vi "VNA and Opticool.vi"() -> ()   [LabVIEW 2022 SP3]
uses:
  <vilib>/Analysis/baseanly.llb/Mean (DBL).vi
  <vilib>/Utility/file.llb/Write Delimited Spreadsheet (DBL).vi
  <vilib>/Analysis/NI_AALBase.lvlib
  Agilent ENA Series/Agilent ENA Series.lvlib
panel:
  in  "stop":bool
  in  "file path (dialog if empty) Scan 2":path=path "C:/Users/B1172_SHG/Documents/NOEMS/test.txt"
  in  "Second Scan":bool
  in  "Port ( 1)  2":i32=1
  in  "Measurement Parameters   2":u16(ring)=1 items=["S11", "S21", "S31", "S41", "S12", "S22", "S32", "S42", "S13", "S23", "S33", "S43", "S14", "S24", "S34", "S44", "A", "B", "C", "D", "R1", "R2", "R3", "R4"]
  in  "Power Level (dBm)  2":dbl=-5.0 format="%^.2g"
  in  "VNA Points  2":i32=1000
  in  "Start (Mhz)  2":dbl=1.0 format="%^.2e"
  in  "Stop (MHz)  2":dbl=10.0 format="%^.2e"
  in  "Trigger Source   2":u16(ring) items=["Internal", "External", "Manual", "BUS"]
  in  "Point Trigger (F: Disable) 3":bool
  in  "Continuous Sweep (T: Enable)  2":bool=TRUE
  in  "Averaging State (F: Off) 3":bool
  in  "Average Factor (16) 3":i32=16
  in  "IF Bandwidth (100000.0)  2":dbl=1000.0 format="%^.1e"
  in  "Smoothing State (F: Off) 3":bool
  in  "Wait time (ms)  2":dbl=4000.0
  out "XY Graph 3":cluster{dbl[], "Primary / Real":dbl[]}(graph)
  in  "Continue":bool
  in  "Field Set when finsihed":dbl
  in  "Port ( 1)":i32=1
  in  "Measurement Parameters":u16(ring)=1 items=["S11", "S21", "S31", "S41", "S12", "S22", "S32", "S42", "S13", "S23", "S33", "S43", "S14", "S24", "S34", "S44", "A", "B", "C", "D", "R1", "R2", "R3", "R4"]
  in  "Power Level (dBm)":dbl=-5.0 format="%^.2g"
  in  "VNA Points":i32=1000
  in  "Start (Mhz)":dbl=1.0 format="%^.2e"
  in  "Stop (MHz)":dbl=10.0 format="%^.2e"
  in  "Trigger Source":u16(ring) items=["Internal", "External", "Manual", "BUS"]
  in  "Point Trigger (F: Disable) 2":bool
  in  "Continuous Sweep (T: Enable)":bool=TRUE
  in  "Averaging State (F: Off) 2":bool
  in  "Average Factor (16) 2":i32=16
  in  "IF Bandwidth (100000.0)":dbl=1000.0 format="%^.1e"
  in  "Smoothing State (F: Off) 2":bool
  in  "Wait time (ms)":dbl=4000.0
  out "XY Graph 2":cluster{dbl[], "Primary / Real":dbl[]}(graph)
  in  "T scan waiting time (min)":dbl=20.0
  in  "Scan T":bool=TRUE
  in  "T Step Size":dbl
  in  "Start B":dbl
  in  "B Step Size":dbl
  in  "B Number of Step":i32=1
  in  "Start T":dbl
  in  "T Number of Step":i32=1
  in  "Temperature Set when finish":dbl=120.0
  in  "file path (dialog if empty)":path=path "C:/Users/B1172_SHG/Documents/NOEMS/test.txt"
  in  "VISA resource name":refnum<visa-resource-name>
  in  "Remote":bool=TRUE
  in  "IP Address":string="169.254.170.239"
  out "Measuring":bool
  out "Temperature":dbl
  in  "WaitForTemperature":bool=TRUE
  in  "WaitForField":bool=TRUE
  in  "Delay":dbl=5.0
  out "Field":dbl
  out "Field\nStatus":i32(ring) items=["MagnetUnknown"=0, "StablePersistent"=1, "WarmingSwitch"=2, "CoolingSwitch"=3, "StableDriven"=4, "Iterating"=5, "Charging"=6, "Discharging"=7, "CurrentError"=8, "MagnetFailure"=15]
  out "Temperature\nStatus":i32(ring) items=["TemperatureUnknown"=0, "Stable"=1, "Tracking"=2, "Near"=5, "Chasing"=6, "Filling"=7, "Standby"=10, "Disabled"=13, "ImpedanceNotFunction"=14, "TempFailure"=15]
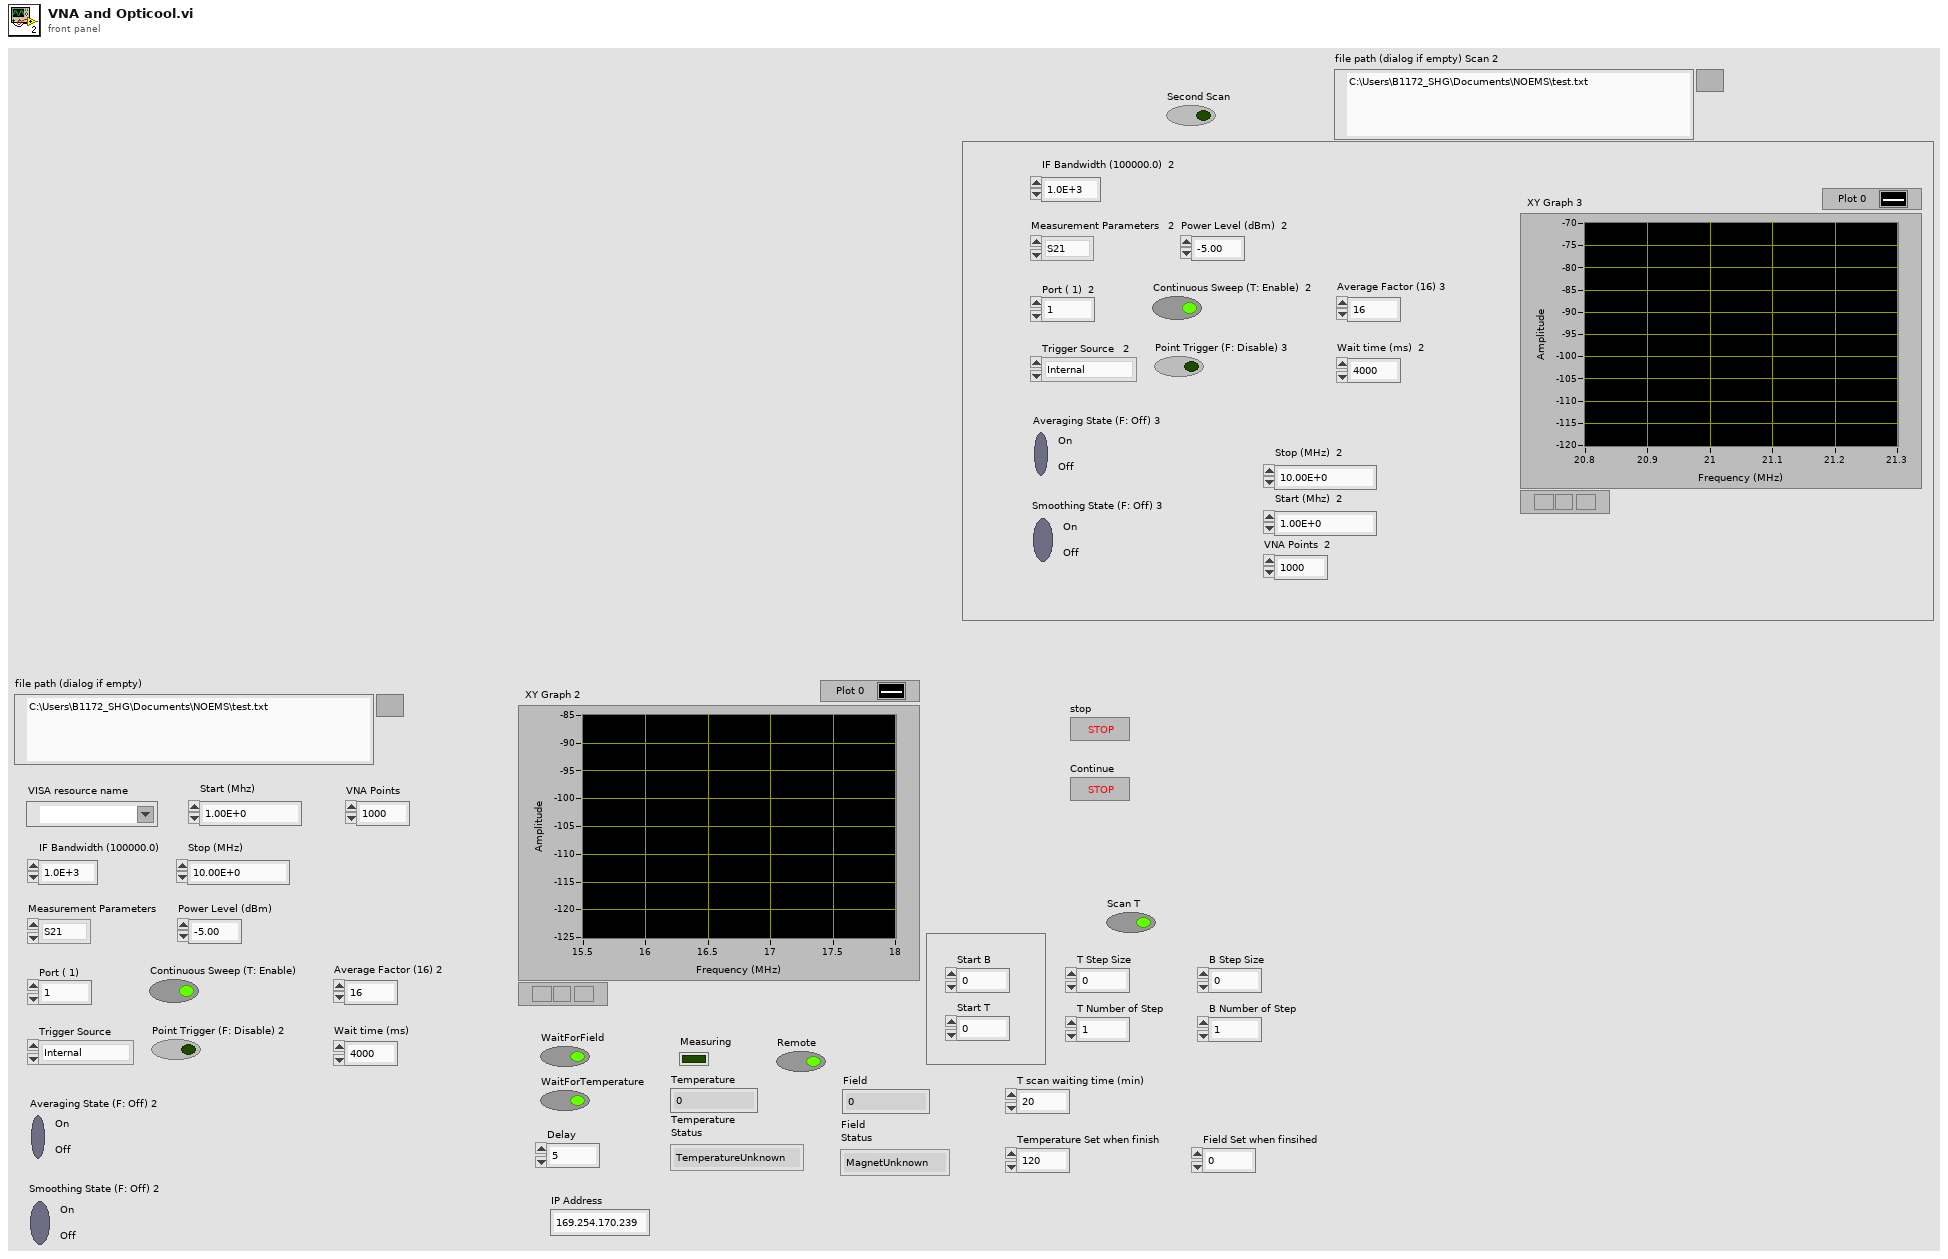
[diagram p1: front panel]
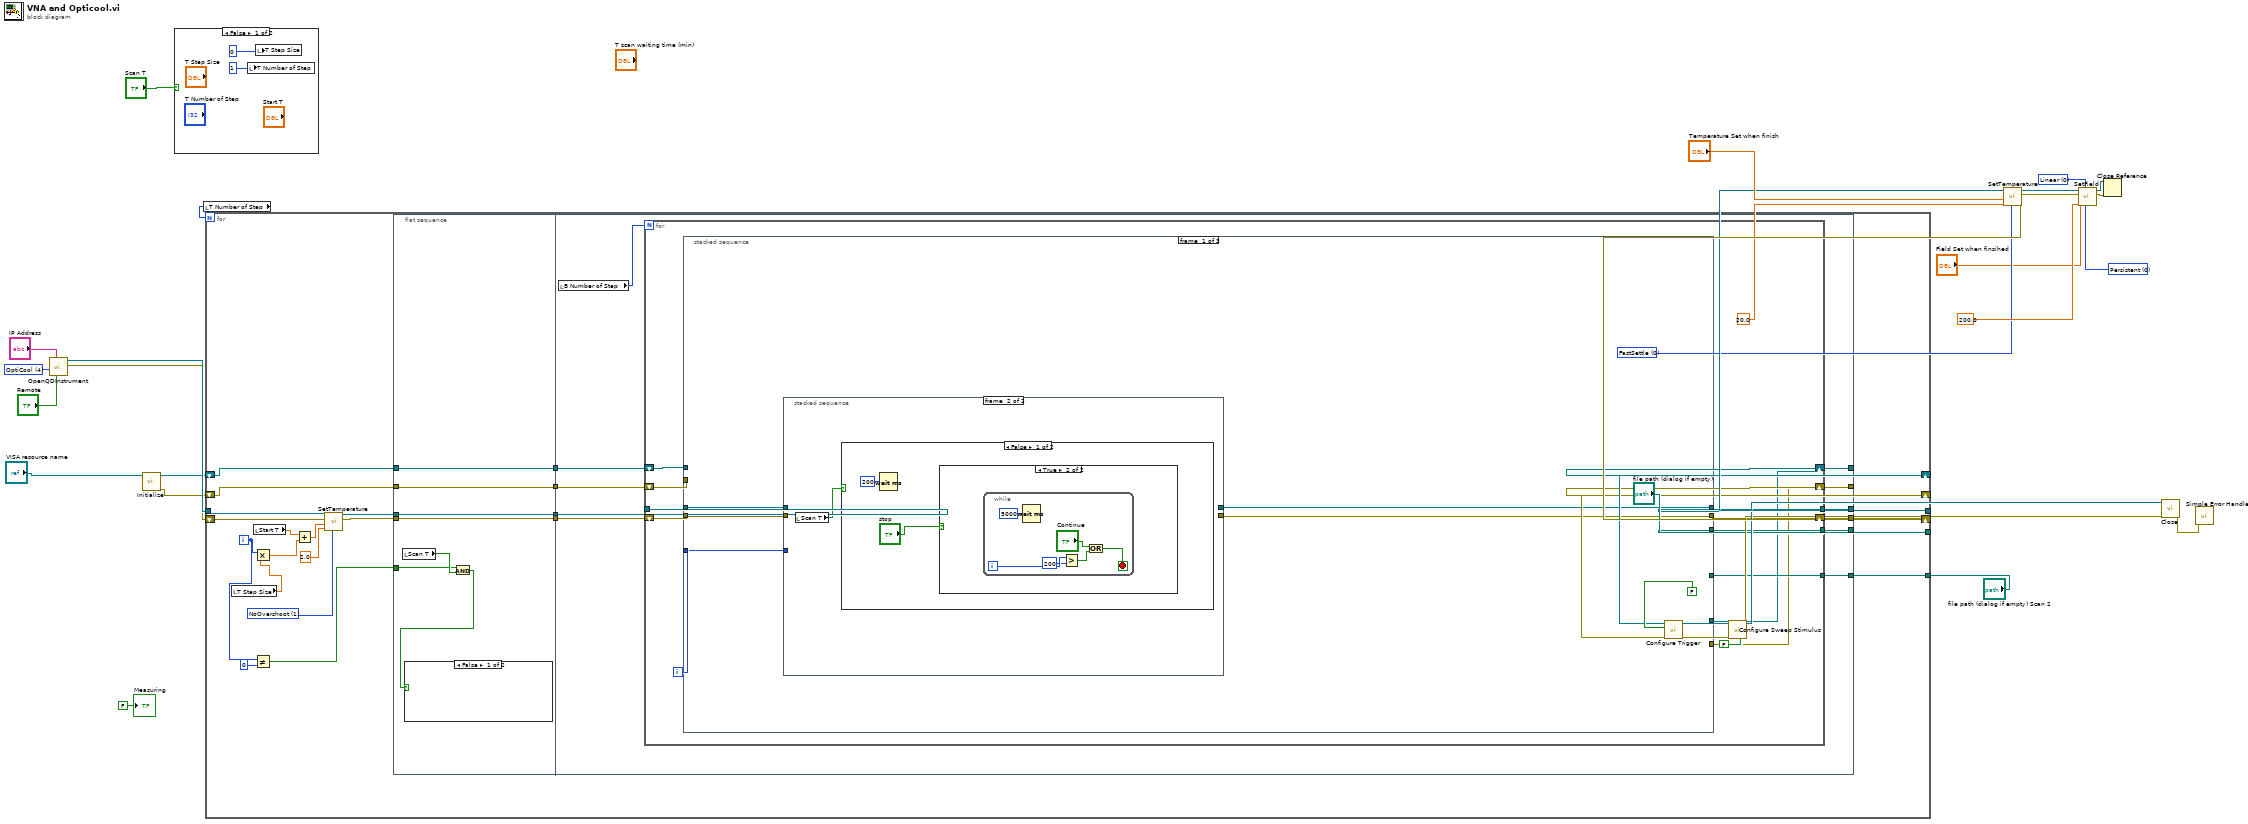
[diagram p0: block diagram]
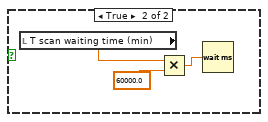
[diagram p2: hidden frame]
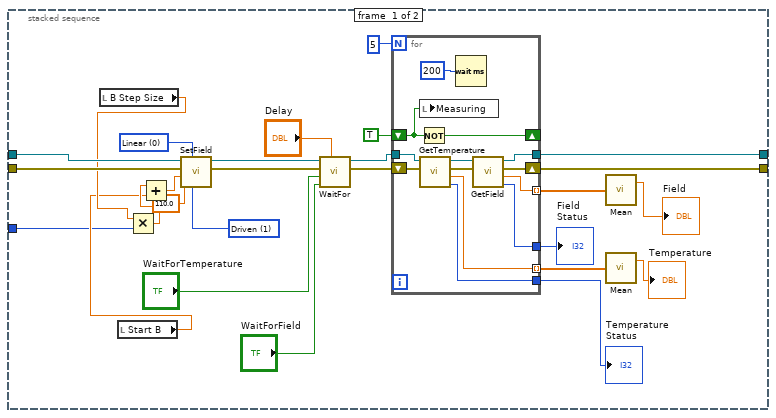
[diagram p3: hidden frame]
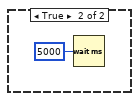
[diagram p5: hidden frame]
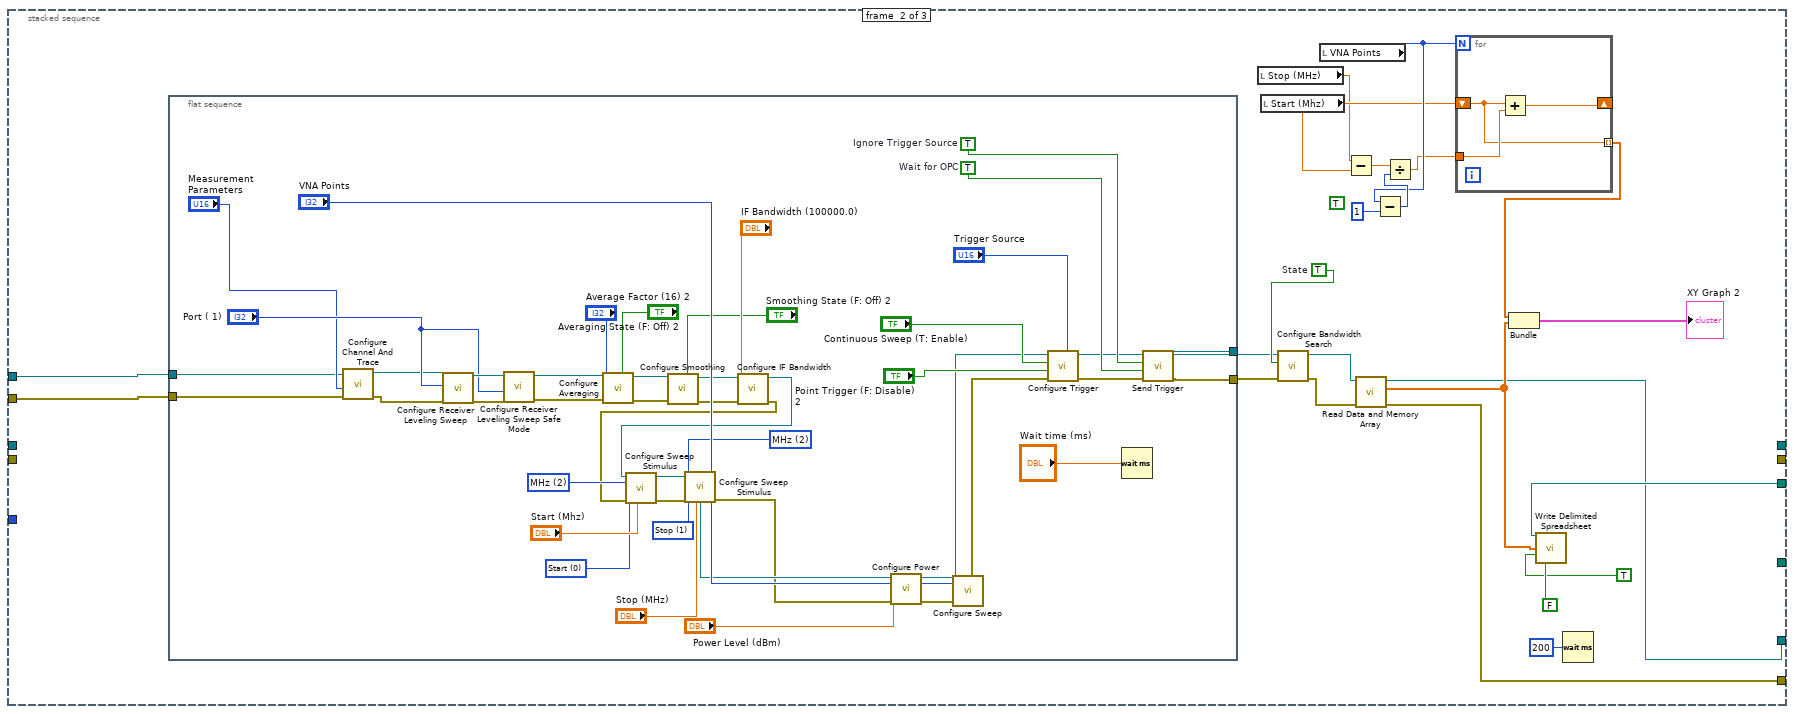
[diagram p6: hidden frame]
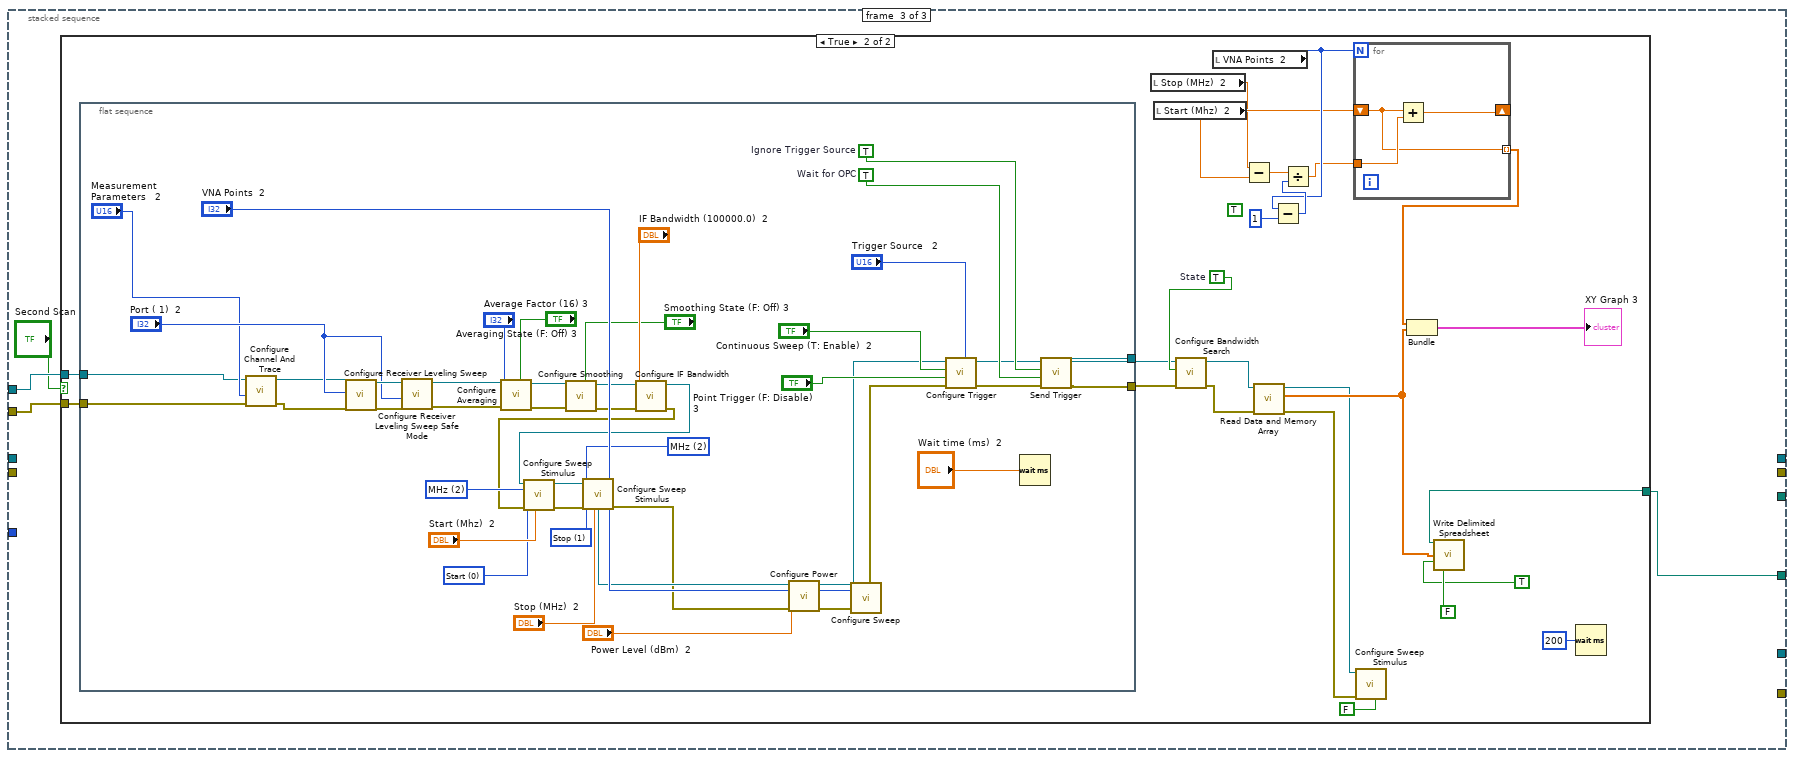
[diagram p7: hidden frame]
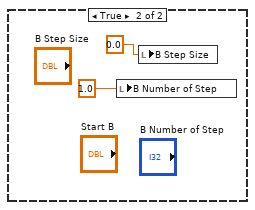
[diagram p9: hidden frame]
diagram:
  w18 = 0 items=["FastSettle", "NoOvershoot"] ("Approach")
  w21 = 4 items=["PPMS", "VersaLab", "DynaCool", "SVSM", "OptiCool"] ("InstrumentType")
  w33 = 0 items=["Persistent", "Driven"] ("Mode")
  w32 = 0 items=["Linear", "NoOvershoot", "Oscillate"] ("Approach")
  n1 = call "OpenQDInstrument.vi"("Remote"="Remote", "IP Address"="IP Address", "InstrumentType"=w21) -> ("error out"=w19:errorcluster, "Instrument Ref"=w20:refnum<k24>)  [unwired: 5 in]
  n2 = call "Initialize.vi"("VISA resource name"="VISA resource name") -> ("error out"=w3:errorcluster, "VISA resource name out"=w5:refnum<visa-resource-name>)  [unwired: 9 in]
  n3 = case shown="False" "Scan T" {
    frame False {
      n4 = local write "T Number of Step"(1) -> ()
      n5 = local write "T Step Size"(0) -> ()
    }
    frame True {
      n6 = local write "B Number of Step"(1.0 ("B Step Size")) -> ()
      n7 = local write "B Step Size"(0.0 ("B Step Size")) -> ()
    }
  }
  n8 = local read "T Number of Step"() -> (w8:i32)
  n9 = for {
    N: w8 -> [_]
    shift-right: [w58] -> w27
    shift-left: w19 -> [w62]
    tunnel: w20 -> [w61]
    tunnel: [w56] -> w24
    tunnel: "file path (dialog if empty)" -> [w52]
    shift-right: [w51] -> w7
    shift-left: w5 -> [w49]
    shift-right: [w50] -> w4
    shift-left: w3 -> [w48]
    tunnel: "file path (dialog if empty) Scan 2" -> [w43]
    i -> [w42]
    w57 = 1 items=["FastSettle", "NoOvershoot"] ("Approach")
    n10 = local read "T Step Size"() -> (w53:dbl)
    n11 = local read "Start T"() -> (w54:dbl)
    n12 = Multiply(x=w42, y=w53) -> (x*y=w55:dbl)
    n13 = Not Equal?(x=w42, y=0) -> (x != y?=w40:bool)
    n14 = Add(x=w54, y=w55) -> (x+y=w64:dbl)
    n15 = call "SetTemperature.vi"("Approach"=w57, "Rate"=2.0, "Temperature"=w64, "error in (no error)"=w62, "Instrument Ref In"=w61) -> ("error out"=w59:errorcluster, "Instrument Ref Out"=w60:refnum<k24>)  [unwired: 2 in, 1 out]
    n16 = flat-sequence {
      tunnel: w48 -> [w68]
      tunnel: w49 -> [w69]
      tunnel: w59 -> [w70]
      tunnel: w60 -> [w71]
      tunnel: [w71] -> w47
      tunnel: [w70] -> w46
      tunnel: [w69] -> w45
      tunnel: [w68] -> w44
      tunnel: w40 -> [w66]
      tunnel: [w83] -> w58
      tunnel: [w82] -> w56
      tunnel: w52 -> [w80]
      tunnel: [w79] -> w51
      tunnel: [w78] -> w50
      tunnel: w47 -> [w85]
      tunnel: w46 -> [w84]
      tunnel: w45 -> [w77]
      tunnel: w44 -> [w76]
      tunnel: w43 -> [w75]
      frame #0 {
        n17 = local read "Scan T"() -> (w67:bool)
        n18 = And(x=w66, y=w67) -> (x .and. y?=w65:bool)
        n19 = case shown="False" w65 {
          frame False {
          }
          frame True {
            n20 = local read "T scan waiting time (min)"() -> (w73:dbl)
            n21 = Multiply(x=w73, y=60000.0) -> (x*y=w72:dbl)
            n22 = Wait (ms)(milliseconds to wait=w72) -> ()  [unwired: 1 out]
          }
        }
      }
      frame #1 {
        n23 = local read "B Number of Step"() -> (w81:i32)
        n24 = for {
          N: w81 -> [_]
          tunnel: w85 -> [w96]
          shift-right: [w93] -> w83
          shift-left: w84 -> [w95]
          tunnel: [w94] -> w82
          tunnel: w80 -> [w92]
          shift-right: [w87] -> w79
          shift-left: w77 -> [w91]
          shift-right: [w86] -> w78
          shift-left: w76 -> [w90]
          tunnel: w75 -> [w88]
          i -> [w89]
          n25 = stacked-sequence {
            tunnel: w96 -> [w101 _ _]
            tunnel: w95 -> [w100 _ _]
            tunnel: [w99 _ _] -> w94
            tunnel: [w98 _ _] -> w93
            tunnel: w92 -> [_ w156 _]
            tunnel: [_ w155 _] -> w87
            tunnel: w91 -> [_ w154 w227]
            tunnel: w90 -> [_ w153 w226]
            tunnel: w89 -> [w97 _ _]
            tunnel: w88 -> [_ _ w224]
            tunnel: [_ w152 _] -> w86
            frame #0 {
              n26 = stacked-sequence {
                tunnel: w101 -> [w123 _]
                tunnel: w100 -> [w122 _]
                tunnel: [w115 _] -> w99
                tunnel: [w112 _] -> w98
                tunnel: w97 -> [w102 _]
                frame #0 {
                  w127 = 0 items=["Linear", "NoOvershoot", "Oscillate"] ("Approach")
                  w128 = 1 items=["Persistent", "Driven"] ("Mode")
                  n27 = local read "B Step Size"() -> (w107:dbl)
                  n28 = local read "Start B"() -> (w104:dbl)
                  n29 = Multiply(x=w107, y=w102) -> (x*y=w106:dbl)
                  n30 = Add(x=w106, y=w104) -> (x+y=w105:dbl)
                  n31 = call "SetField.vi"("Mode"=w128, "Approach"=w127, "Rate"=110.0, "Field"=w105, "error in (no error)"=w122, "Instrument Ref In"=w123) -> ("error out"=w121:errorcluster, "Instrument Ref Out"=w117:refnum<k24>)  [unwired: 1 in, 1 out]
                  n32 = call "WaitFor.vi"("Delay"="Delay", "Wait For Field"="WaitForField", "Wait For Temperature"="WaitForTemperature", "error in (no error)"=w121, "Instrument Ref In"=w117) -> ("error out"=w126:errorcluster, "Instrument Ref Out"=w116:refnum<k24>)  [unwired: 5 in]
                  n33 = for {
                    N: 5 -> [_]
                    shift-right: [w141] -> _
                    shift-left: TRUE -> [w139]
                    shift-right: [w136] -> w112
                    shift-left: w126 -> [w138]
                    tunnel: w116 -> [w135]
                    tunnel: [w133] -> w115
                    tunnel: [w130] -> w114
                    tunnel: [w129] -> w113
                    tunnel: [w131] -> w110 mode=indexing
                    tunnel: [w132] -> w111 mode=indexing
                    n34 = Not(x=w139) -> (.not. x?=w141:bool)
                    n35 = local write "Measuring"(w139) -> ()
                    n36 = call "GetTemperature.vi"("error in (no error)"=w138, "Instrument Ref In"=w135) -> ("Temperature\nStatus"=w129:i32, "Temperature"=w132:dbl, "error out"=w137:errorcluster, "Instrument Ref Out"=w134:refnum<k24>)  [unwired: 3 in, 1 out]
                    n37 = Wait (ms)(milliseconds to wait=u32 200) -> ()  [unwired: 1 out]
                    n38 = call "GetField.vi"("error in (no error)"=w137, "Instrument Ref In"=w134) -> ("Field\nStatus"=w130:i32, "Field"=w131:dbl, "error out"=w136:errorcluster, "Instrument Ref Out"=w133:refnum<k24>)  [unwired: 3 in, 1 out]
                  }
                  "Field\nStatus" <- w114
                  "Temperature\nStatus" <- w113
                  n39 = call-poly <vilib>:"Mean.vi"("X"=w110) -> ("mean"=→"Field":dbl)  [unwired: 1 out]
                  n40 = call-poly <vilib>:"Mean.vi"("X"=w111) -> ("mean"=→"Temperature":dbl)  [unwired: 1 out]
                }
                frame #1 {
                  n41 = local read "Scan T"() -> (w142:bool)
                  n42 = case shown="False" w142 {
                    frame False {
                      n43 = Wait (ms)(milliseconds to wait=u32 200) -> ()  [unwired: 1 out]
                      n44 = case shown="True" "stop" {
                        frame False {
                        }
                        frame True {
                          n45 = while {
                            i -> [w146]
                            stop <- w148 stop-if-true
                            n46 = Wait (ms)(milliseconds to wait=u32 5000) -> ()  [unwired: 1 out]
                            n47 = Greater?(x=w146, y=200) -> (0:w147:bool)
                            n48 = Or(x="Continue", y=w147) -> (x .or. y?=w148:bool)
                          }
                        }
                      }
                    }
                    frame True {
                      n49 = Wait (ms)(milliseconds to wait=u32 5000) -> ()  [unwired: 1 out]
                    }
                  }
                }
              }
            }
            frame #1 {
              w162 = TRUE  # State
              (unwired) TRUE ("Continuous Sweep (T: Enable)")
              n50 = flat-sequence {
                tunnel: [w178] -> w159
                tunnel: [w177] -> w158
                tunnel: w154 -> [w176]
                tunnel: w153 -> [w175]
                frame #0 {
                  w204 = u16 2 items=["Hz", "kHz", "MHz", "GHz", "dBm", "s", "V"] ("Unit (0: Hz)")
                  w205 = u16 2 items=["Hz", "kHz", "MHz", "GHz", "dBm", "s", "V"] ("Unit (0: Hz)")
                  w206 = u16 1 items=["Start", "Stop", "Center", "Span"] ("Stimulus (0: Start)")
                  w207 = u16 0 items=["Start", "Stop", "Center", "Span"] ("Stimulus (0: Start)")
                  w219 = TRUE  # Wait for OPC
                  w220 = TRUE  # Ignore Trigger Source
                  n51 = call "Configure Channel And Trace.vi"("error in (no error)"=w175, "Measurement Parameters (0: S11)"="Measurement Parameters", "VISA resource name"=w176) -> ("error out"=w190:errorcluster, "VISA resource name out"=w193:refnum<visa-resource-name>)  [unwired: 7 in]
                  n52 = call "Configure Receiver Leveling Sweep.vi"("VISA resource name"=w193, "Port ( 1)"="Port ( 1)", "error in (no error)"=w190) -> ("VISA resource name out"=w217:refnum<visa-resource-name>, "error out"=w189:errorcluster)  [unwired: 15 in]
                  n53 = call "Configure Receiver Leveling Sweep Safe Mode.vi"("error in (no error)"=w189, "Port ( 1)"="Port ( 1)", "VISA resource name"=w217) -> ("error out"=w188:errorcluster, "VISA resource name out"=w192:refnum<visa-resource-name>)  [unwired: 7 in]
                  n54 = call "Configure Averaging.vi"("Averaging State (F: Off)"="Averaging State (F: Off) 2", "error in (no error)"=w188, "Factor (16)"="Average Factor (16) 2", "VISA resource name"=w192) -> ("error out"=w187:errorcluster, "VISA resource name out"=w200:refnum<visa-resource-name>)  [unwired: 6 in]
                  n55 = call "Configure Smoothing.vi"("Smoothing State (F: Off)"="Smoothing State (F: Off) 2", "error in (no error)"=w187, "VISA resource name"=w200) -> ("error out"=w186:errorcluster, "VISA resource name out"=w199:refnum<visa-resource-name>)  [unwired: 7 in]
                  n56 = call "Configure IF Bandwidth.vi"("error in (no error)"=w186, "IF Bandwidth (100000.0)"="IF Bandwidth (100000.0)", "VISA resource name"=w199) -> ("error out"=w185:errorcluster, "VISA resource name out"=w198:refnum<visa-resource-name>)  [unwired: 7 in]
                  n57 = call "Configure Sweep Stimulus.vi"("Parameter (0.0)"="Start (Mhz)", "error in (no error)"=w185, "Stimulus (0: Start)"=w207, "Unit (0: Hz)"=w205, "VISA resource name"=w198) -> ("error out"=w184:errorcluster, "VISA resource name out"=w211:refnum<visa-resource-name>)  [unwired: 5 in]
                  n58 = call "Configure Sweep Stimulus.vi"("Parameter (0.0)"="Stop (MHz)", "error in (no error)"=w184, "Stimulus (0: Start)"=w206, "Unit (0: Hz)"=w204, "VISA resource name"=w211) -> ("error out"=w183:errorcluster, "VISA resource name out"=w210:refnum<visa-resource-name>)  [unwired: 5 in]
                  n59 = call "Configure Power.vi"("VISA resource name"=w210, "Power Level (0.0)"="Power Level (dBm)", "error in (no error)"=w183) -> ("VISA resource name out"=w213:refnum<visa-resource-name>, "error out"=w182:errorcluster)  [unwired: 11 in]
                  n60 = call "Configure Sweep.vi"("VISA resource name"=w213, "Number of Measurement Points (201)"="VNA Points", "error in (no error)"=w182) -> ("VISA resource name out"=w191:refnum<visa-resource-name>, "error out"=w181:errorcluster)  [unwired: 11 in]
                  n61 = call "Configure Trigger.vi"("Trigger Source (0: Internal)"="Trigger Source", "error in (no error)"=w181, "Point Trigger (F: Disable)"="Point Trigger (F: Disable) 2", "Continuous Sweep (T: Enable)"="Continuous Sweep (T: Enable)", "VISA resource name"=w191) -> ("error out"=w180:errorcluster, "VISA resource name out"=w218:refnum<visa-resource-name>)  [unwired: 5 in]
                  n62 = Wait (ms)(milliseconds to wait="Wait time (ms)") -> ()  [unwired: 1 out]
                  n63 = call "Send Trigger.vi"("error in (no error)"=w180, "Wait for OPC (F: Do not Wait)"=w219, "Ignore Trigger Source (F: Do not Ignore)"=w220, "VISA resource name"=w218) -> ("error out"=w177:errorcluster, "VISA resource name out"=w178:refnum<visa-resource-name>)  [unwired: 6 in]
                }
              }
              n64 = local read "Stop (MHz)"() -> (w167:dbl)
              n65 = local read "Start (Mhz)"() -> (w168:dbl)
              n66 = call "Configure Bandwidth Search.vi"("error in (no error)"=w158, "Result Display State (F: Disable)"=w162, "VISA resource name"=w159) -> ("error out"=w160:errorcluster, "VISA resource name out"=w161:refnum<visa-resource-name>)  [unwired: 7 in]
              n67 = local read "VNA Points"() -> (w171:i32)
              n68 = Subtract(x=w167, y=w168) -> (x-y=w169:dbl)
              n69 = call "Read Data and Memory Array.vi"("error in (no error)"=w160, "VISA resource name"=w161) -> ("error out"=w152:errorcluster, "Primary / Real"=w157:dbl[], "VISA resource name out"=w155:refnum<visa-resource-name>)  [unwired: 6 in, 1 out]
              n70 = Subtract(x=w171, y=1) -> (x-y=w172:i32)
              n71 = Divide(x=w169, y=w172) -> (x/y=w170:dbl)
              n72 = for {
                N: w171 -> [_]
                shift-right: [w223] -> _
                shift-left: w168 -> [w221]
                tunnel: w170 -> [w222]
                tunnel: [w221] -> w165 mode=indexing
                n73 = Add(x=w221, y=w222) -> (x+y=w223:dbl)
              }
              n74 = Bundle(w165, "Primary / Real"=w157) -> (→"XY Graph 2":cluster{dbl[], "Primary / Real":dbl[]})  [unwired: 1 in]
              n75 = call-poly <vilib>:"Write Delimited Spreadsheet.vi"("file path (dialog if empty)"=w156, "1D data"=w157, "append to file? (new file:F)"=TRUE, "transpose? (no:F)"=FALSE) -> ()  [unwired: 10 in, 2 out]
              n76 = Wait (ms)(milliseconds to wait=u32 200) -> ()  [unwired: 1 out]
            }
            frame #2 {
              n77 = case shown="True" "Second Scan" {
                tunnel: w227 -> [_ w233]
                tunnel: w226 -> [_ w232]
                tunnel: w224 -> [_ w231]
                frame False {
                }
                frame True {
                  w239 = TRUE  # State
                  (unwired) TRUE ("Continuous Sweep (T: Enable)")
                  n78 = flat-sequence {
                    tunnel: [w255] -> w236
                    tunnel: [w254] -> w235
                    tunnel: w233 -> [w253]
                    tunnel: w232 -> [w252]
                    frame #0 {
                      w281 = u16 2 items=["Hz", "kHz", "MHz", "GHz", "dBm", "s", "V"] ("Unit (0: Hz)")
                      w282 = u16 2 items=["Hz", "kHz", "MHz", "GHz", "dBm", "s", "V"] ("Unit (0: Hz)")
                      w283 = u16 1 items=["Start", "Stop", "Center", "Span"] ("Stimulus (0: Start)")
                      w284 = u16 0 items=["Start", "Stop", "Center", "Span"] ("Stimulus (0: Start)")
                      w296 = TRUE  # Wait for OPC
                      w297 = TRUE  # Ignore Trigger Source
                      n79 = call "Configure Channel And Trace.vi"("error in (no error)"=w252, "Measurement Parameters (0: S11)"="Measurement Parameters   2", "VISA resource name"=w253) -> ("error out"=w267:errorcluster, "VISA resource name out"=w270:refnum<visa-resource-name>)  [unwired: 7 in]
                      n80 = call "Configure Receiver Leveling Sweep.vi"("VISA resource name"=w270, "Port ( 1)"="Port ( 1)  2", "error in (no error)"=w267) -> ("VISA resource name out"=w294:refnum<visa-resource-name>, "error out"=w266:errorcluster)  [unwired: 15 in]
                      n81 = call "Configure Receiver Leveling Sweep Safe Mode.vi"("error in (no error)"=w266, "Port ( 1)"="Port ( 1)  2", "VISA resource name"=w294) -> ("error out"=w265:errorcluster, "VISA resource name out"=w269:refnum<visa-resource-name>)  [unwired: 7 in]
                      n82 = call "Configure Averaging.vi"("Averaging State (F: Off)"="Averaging State (F: Off) 3", "error in (no error)"=w265, "Factor (16)"="Average Factor (16) 3", "VISA resource name"=w269) -> ("error out"=w264:errorcluster, "VISA resource name out"=w277:refnum<visa-resource-name>)  [unwired: 6 in]
                      n83 = call "Configure Smoothing.vi"("Smoothing State (F: Off)"="Smoothing State (F: Off) 3", "error in (no error)"=w264, "VISA resource name"=w277) -> ("error out"=w263:errorcluster, "VISA resource name out"=w276:refnum<visa-resource-name>)  [unwired: 7 in]
                      n84 = call "Configure IF Bandwidth.vi"("error in (no error)"=w263, "IF Bandwidth (100000.0)"="IF Bandwidth (100000.0)  2", "VISA resource name"=w276) -> ("error out"=w262:errorcluster, "VISA resource name out"=w275:refnum<visa-resource-name>)  [unwired: 7 in]
                      n85 = call "Configure Sweep Stimulus.vi"("Parameter (0.0)"="Start (Mhz)  2", "error in (no error)"=w262, "Stimulus (0: Start)"=w284, "Unit (0: Hz)"=w282, "VISA resource name"=w275) -> ("error out"=w261:errorcluster, "VISA resource name out"=w288:refnum<visa-resource-name>)  [unwired: 5 in]
                      n86 = call "Configure Sweep Stimulus.vi"("Parameter (0.0)"="Stop (MHz)  2", "error in (no error)"=w261, "Stimulus (0: Start)"=w283, "Unit (0: Hz)"=w281, "VISA resource name"=w288) -> ("error out"=w260:errorcluster, "VISA resource name out"=w287:refnum<visa-resource-name>)  [unwired: 5 in]
                      n87 = call "Configure Power.vi"("VISA resource name"=w287, "Power Level (0.0)"="Power Level (dBm)  2", "error in (no error)"=w260) -> ("VISA resource name out"=w290:refnum<visa-resource-name>, "error out"=w259:errorcluster)  [unwired: 11 in]
                      n88 = call "Configure Sweep.vi"("VISA resource name"=w290, "Number of Measurement Points (201)"="VNA Points  2", "error in (no error)"=w259) -> ("VISA resource name out"=w268:refnum<visa-resource-name>, "error out"=w258:errorcluster)  [unwired: 11 in]
                      n89 = call "Configure Trigger.vi"("Trigger Source (0: Internal)"="Trigger Source   2", "error in (no error)"=w258, "Point Trigger (F: Disable)"="Point Trigger (F: Disable) 3", "Continuous Sweep (T: Enable)"="Continuous Sweep (T: Enable)  2", "VISA resource name"=w268) -> ("error out"=w257:errorcluster, "VISA resource name out"=w295:refnum<visa-resource-name>)  [unwired: 5 in]
                      n90 = Wait (ms)(milliseconds to wait="Wait time (ms)  2") -> ()  [unwired: 1 out]
                      n91 = call "Send Trigger.vi"("error in (no error)"=w257, "Wait for OPC (F: Do not Wait)"=w296, "Ignore Trigger Source (F: Do not Ignore)"=w297, "VISA resource name"=w295) -> ("error out"=w254:errorcluster, "VISA resource name out"=w255:refnum<visa-resource-name>)  [unwired: 6 in]
                    }
                  }
                  n92 = local read "Stop (MHz)  2"() -> (w244:dbl)
                  n93 = local read "Start (Mhz)  2"() -> (w245:dbl)
                  n94 = call "Configure Bandwidth Search.vi"("error in (no error)"=w235, "Result Display State (F: Disable)"=w239, "VISA resource name"=w236) -> ("error out"=w237:errorcluster, "VISA resource name out"=w238:refnum<visa-resource-name>)  [unwired: 7 in]
                  n95 = local read "VNA Points  2"() -> (w248:i32)
                  n96 = Subtract(x=w244, y=w245) -> (x-y=w246:dbl)
                  n97 = call "Read Data and Memory Array.vi"("error in (no error)"=w237, "VISA resource name"=w238) -> ("error out"=w230:errorcluster, "Primary / Real"=w234:dbl[], "VISA resource name out"=w229:refnum<visa-resource-name>)  [unwired: 6 in, 1 out]
                  n98 = Subtract(x=w248, y=1) -> (x-y=w249:i32)
                  n99 = Divide(x=w246, y=w249) -> (x/y=w247:dbl)
                  n100 = for {
                    N: w248 -> [_]
                    shift-right: [w300] -> _
                    shift-left: w245 -> [w298]
                    tunnel: w247 -> [w299]
                    tunnel: [w298] -> w242 mode=indexing
                    n101 = Add(x=w298, y=w299) -> (x+y=w300:dbl)
                  }
                  n102 = call "Configure Sweep Stimulus.vi"("Signal Output (T: On)"=FALSE, "error in (no error)"=w230, "VISA resource name"=w229) -> ()  [unwired: 7 in, 2 out]
                  n103 = Bundle(w242, "Primary / Real"=w234) -> (→"XY Graph 3":cluster{dbl[], "Primary / Real":dbl[]})  [unwired: 1 in]
                  n104 = call-poly <vilib>:"Write Delimited Spreadsheet.vi"("file path (dialog if empty)"=w231, "1D data"=w234, "append to file? (new file:F)"=TRUE, "transpose? (no:F)"=FALSE) -> ()  [unwired: 10 in, 2 out]
                  n105 = Wait (ms)(milliseconds to wait=u32 200) -> ()  [unwired: 1 out]
                }
              }
            }
          }
        }
      }
    }
  }
  n106 = call "Configure Trigger.vi"("error in (no error)"=w4, "Continuous Sweep (T: Enable)"=FALSE, "VISA resource name"=w7) -> ("error out"=w12:errorcluster, "VISA resource name out"=w13:refnum<visa-resource-name>)  [unwired: 7 in]
  n107 = call "Configure Sweep Stimulus.vi"("Signal Output (T: On)"=FALSE, "error in (no error)"=w12, "VISA resource name"=w13) -> ("error out"=w15:errorcluster, "VISA resource name out"=w16:refnum<visa-resource-name>)  [unwired: 7 in]
  n108 = call "SetTemperature.vi"("Approach"=w18, "Rate"=20.0, "Temperature"="Temperature Set when finish", "error in (no error)"=w27, "Instrument Ref In"=w24) -> ("error out"=w30:errorcluster, "Instrument Ref Out"=w29:refnum<k24>)  [unwired: 2 in, 1 out]
  n109 = call "SetField.vi"("Mode"=w33, "Approach"=w32, "Rate"=200.0, "Field"="Field Set when finsihed", "error in (no error)"=w30, "Instrument Ref In"=w29) -> ("error out"=w35:errorcluster, "Instrument Ref Out"=w34:refnum<k24>)  [unwired: 1 in, 1 out]
  n110 = Close Reference(reference=w34, error in (no error)=w35) -> ()  [unwired: 1 out]
  n111 = call "Close.vi"("error in (no error)"=w15, "VISA resource name"=w16) -> ("error out"=w17:errorcluster)  [unwired: 9 in]
  n112 = call <vilib>:"Simple Error Handler.vi"("error in (no error)"=w17) -> ()  [unwired: 4 in, 5 out]
  "Measuring" <- FALSE
